vi "Ping.vi"(8 "Error In":errorcluster, 11 "Test LNA in":refnum<class "TestLNA.lvclass">) -> (0 "Error Out":errorcluster, 3 "Test LNA out":refnum<class "TestLNA.lvclass">)   [LabVIEW 2015, in "TestLNA.lvlib" / "TestLNA.lvclass"]
doc: "Display ping message dialog."
uses:
  TestLNA.lvclass
  CSPP_Core/Actors/CS++BaseActor/CS++BaseActor.lvclass/CS++BaseActor.ctl
  CSPP_Core/Actors/CS++BaseActor/Read Object Name.vi
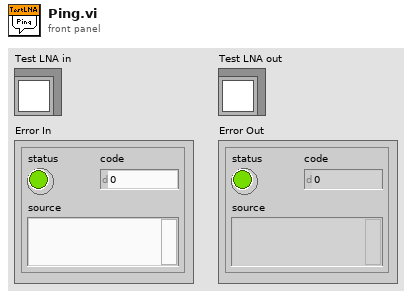
[diagram p1: front panel]
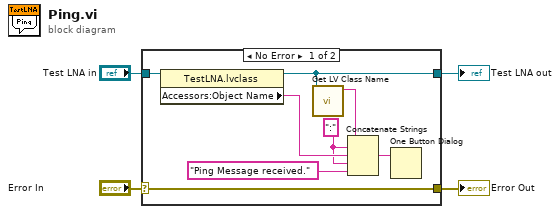
[diagram p0: block diagram]
diagram:
  n1 = case shown="No Error" "Error In" {
    selector: "Error In" -> [w12 w14]
    tunnel: [w12 w14] -> w3
    tunnel: [w7 w13] -> w1
    tunnel: "Test LNA in" -> [w8 w13]
    frame No Error {
      w5 = ":" ("string")
      n2 = property class="TestLNA.lvclass"(reference=w8) -> (reference out=w7:refnum<class "TestLNA.lvclass">, "Accessors:Object Name"=w6:string)  [unwired: 1 in, 1 out]
      n3 = call <vilib>:"Get LV Class Name.vi"("object"=w7) -> ("class name"=w9:string)  [unwired: 9 in, 1 out]
      n4 = Concatenate Strings(w9, w5, w6, w5, "Ping Message received." ("message")) -> (w10:string)
      n5 = One Button Dialog(message=w10) -> ()  [unwired: 1 in, 1 out]
    }
    frame Error {
    }
  }
  "Error Out" <- w3
  "Test LNA out" <- w1
